vi "BuildGraph.vi"() -> (2 "S2":waveform(dbl)[](array[waveform]), 3 "S1":waveform(dbl)[](array[waveform]))   [LabVIEW 2018, in "GUI.lvclass"]
uses:
  GUI.lvclass
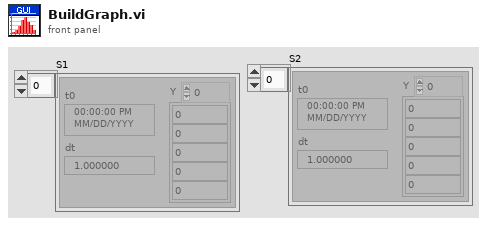
[diagram p1: front panel]
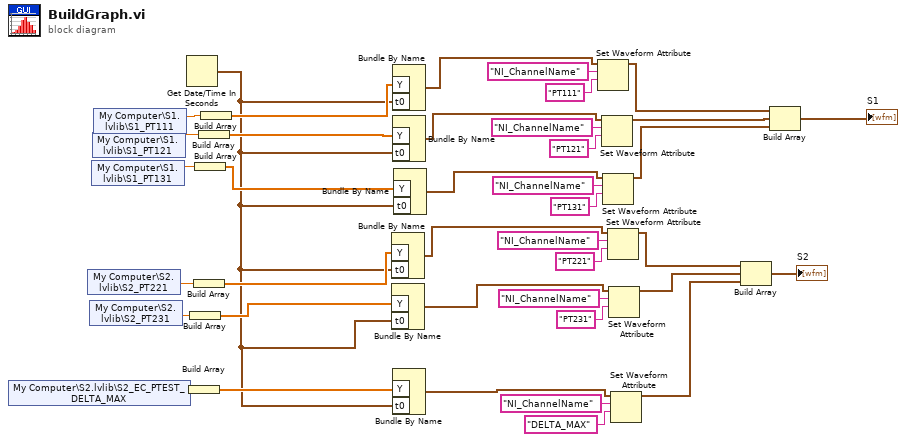
[diagram p0: block diagram]
diagram:
  n1 = shared-variable "My Computer\\S2.lvlib\\S2_EC_PTEST_DELTA_MAX"() -> (w7:dbl)  [unwired: 1 in, 1 out]
  n2 = shared-variable "My Computer\\S2.lvlib\\S2_PT221"() -> (w21:dbl)  [unwired: 1 in, 1 out]
  n3 = shared-variable "My Computer\\S2.lvlib\\S2_PT231"() -> (w20:dbl)  [unwired: 1 in, 1 out]
  n4 = shared-variable "My Computer\\S1.lvlib\\S1_PT131"() -> (w8:dbl)  [unwired: 1 in, 1 out]
  n5 = shared-variable "My Computer\\S1.lvlib\\S1_PT121"() -> (w35:dbl)  [unwired: 1 in, 1 out]
  n6 = shared-variable "My Computer\\S1.lvlib\\S1_PT111"() -> (w34:dbl)  [unwired: 1 in, 1 out]
  n7 = Get Date/Time In Seconds() -> (seconds since 1Jan1904=w5:timestamp)
  n8 = Build Array(w7) -> (w6:dbl[])
  n9 = Build Array(w20) -> (w18:dbl[])
  n10 = Build Array(w21) -> (w19:dbl[])
  n11 = Build Array(w8) -> (w38:dbl[])
  n12 = Build Array(w35) -> (w37:dbl[])
  n13 = Build Array(w34) -> (w36:dbl[])
  n14 = Bundle By Name("Y"=w19, "t0"=w5) -> (w13:waveform(dbl))  [unwired: 1 in]
  n15 = Bundle By Name("Y"=w18, "t0"=w5) -> (w12:waveform(dbl))  [unwired: 1 in]
  n16 = Bundle By Name("Y"=w36, "t0"=w5) -> (w31:waveform(dbl))  [unwired: 1 in]
  n17 = Bundle By Name("Y"=w37, "t0"=w5) -> (w27:waveform(dbl))  [unwired: 1 in]
  n18 = Bundle By Name("Y"=w6, "t0"=w5) -> (w2:waveform(dbl))  [unwired: 1 in]
  n19 = Bundle By Name("Y"=w38, "t0"=w5) -> (w24:waveform(dbl))  [unwired: 1 in]
  n20 = Set Waveform Attribute(5:"PT111" ("name"), 6:"NI_ChannelName" ("name"), 7:w31) -> (3:w30:waveform(dbl))  [unwired: 1 in, 2 out]
  n21 = Set Waveform Attribute(5:"PT121" ("name"), 6:"NI_ChannelName" ("name"), 7:w27) -> (3:w22:waveform(dbl))  [unwired: 1 in, 2 out]
  n22 = Set Waveform Attribute(5:"PT131" ("name"), 6:"NI_ChannelName" ("name"), 7:w24) -> (3:w23:waveform(dbl))  [unwired: 1 in, 2 out]
  n23 = Set Waveform Attribute(5:"PT221" ("name"), 6:"NI_ChannelName" ("name"), 7:w13) -> (3:w11:waveform(dbl))  [unwired: 1 in, 2 out]
  n24 = Set Waveform Attribute(5:"PT231" ("name"), 6:"NI_ChannelName" ("name"), 7:w12) -> (3:w10:waveform(dbl))  [unwired: 1 in, 2 out]
  n25 = Set Waveform Attribute(5:"DELTA_MAX" ("name"), 6:"NI_ChannelName" ("name"), 7:w2) -> (3:w1:waveform(dbl))  [unwired: 1 in, 2 out]
  n26 = Build Array(w11, w10, w1) -> (→"S2":waveform(dbl)[])
  n27 = Build Array(w30, w22, w23) -> (→"S1":waveform(dbl)[])
